vi "compareScan_Read.vi"() -> ()   [LabVIEW 2018]
uses:
  MotorController/#include/Global textParse.vi
panel:
  out "ILpass":bool=TRUE
  out "IRCpass":bool=TRUE
  out "Fpass":bool=TRUE
  out "ILimit":string
  out "IrComp":string
  out "Firmware":string
  out "Test":string
  in  "E-Stop":bool
  in  "Barcode Scan":string
  out "ScanNumber":string
  out "NumberMatch":bool
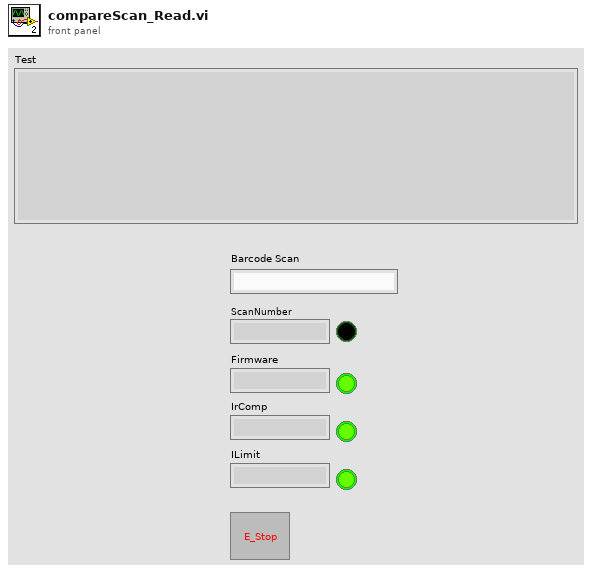
[diagram p1: front panel]
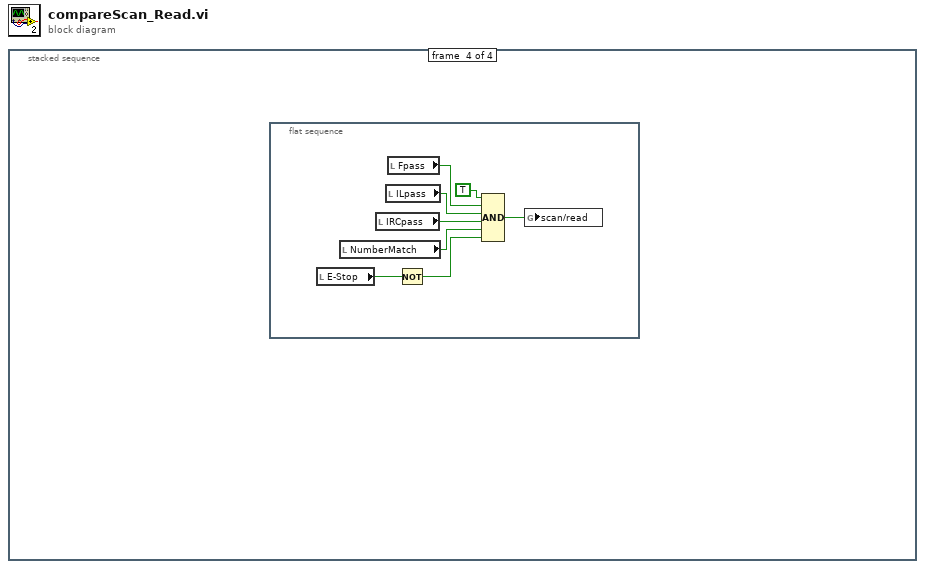
[diagram p0: block diagram]
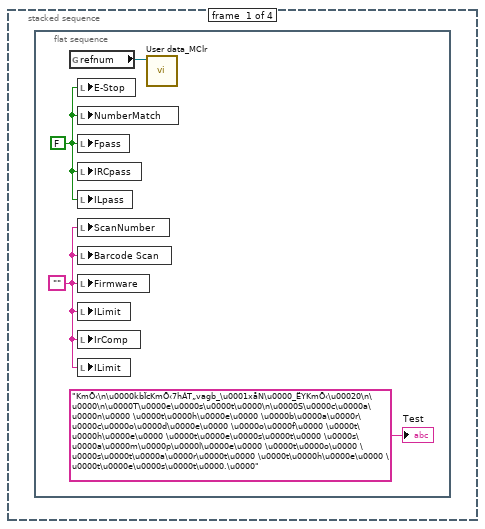
[diagram p2: hidden frame]
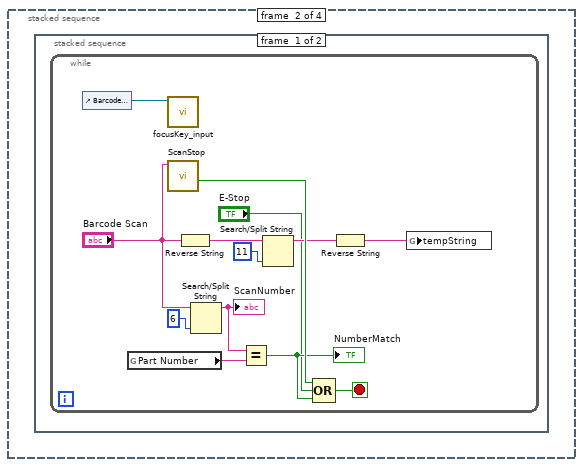
[diagram p3: hidden frame]
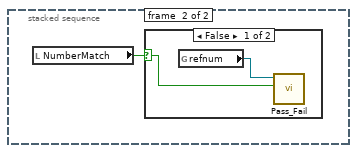
[diagram p4: hidden frame]
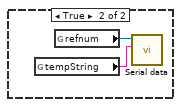
[diagram p5: hidden frame]
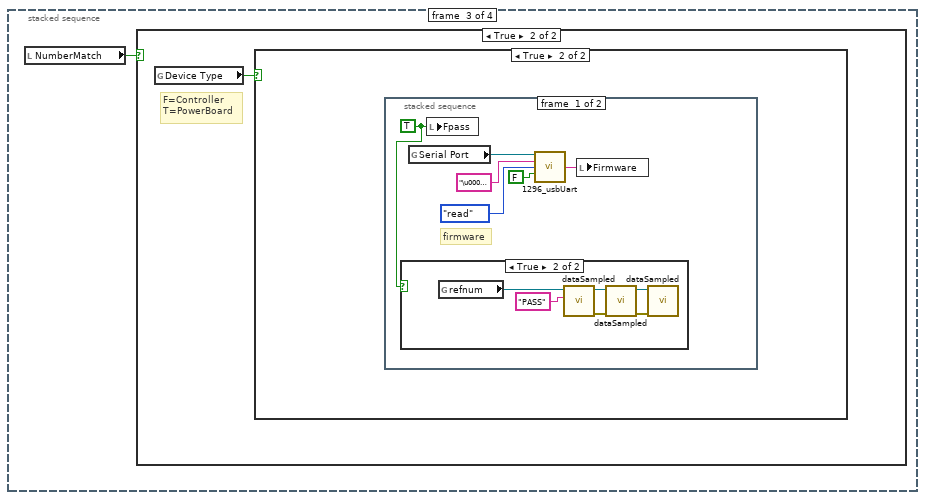
[diagram p6: hidden frame]
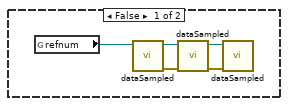
[diagram p7: hidden frame]
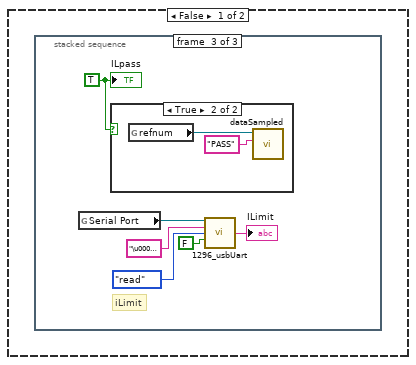
[diagram p8: hidden frame]
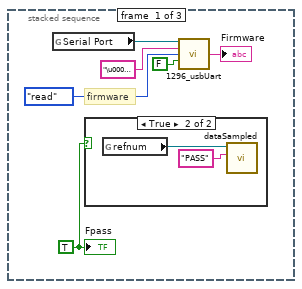
[diagram p9: hidden frame]
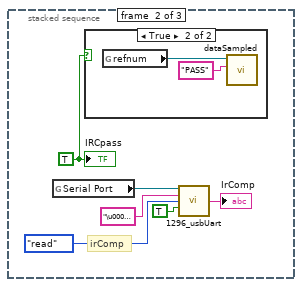
[diagram p11: hidden frame]
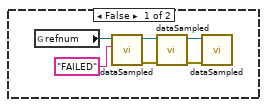
[diagram p14: hidden frame]
diagram:
  n1 = stacked-sequence {
    frame #0 {
      n2 = flat-sequence {
        frame #0 {
          w3 = FALSE
          w2 = ""
          n3 = global read "Global textParse.vi" "refnum"() -> (w4:refnum<file>)
          n4 = local write "E-Stop"(w3) -> ()
          n5 = local write "NumberMatch"(w3) -> ()
          n6 = local write "Fpass"(w3) -> ()
          n7 = local write "IRCpass"(w3) -> ()
          n8 = local write "ILpass"(w3) -> ()
          n9 = local write "ScanNumber"(w2) -> ()
          n10 = local write "Barcode Scan"(w2) -> ()
          n11 = local write "Firmware"(w2) -> ()
          n12 = local write "ILimit"(w2) -> ()
          n13 = local write "IrComp"(w2) -> ()
          n14 = local write "ILimit"(w2) -> ()
          n15 = call "User data_MClr.vi"("refnum in"=w4) -> ()  [unwired: 7 in, 2 out]
          "Test" <- "KmÕ‹\n\u0000kbÏcKmÕ‹7hÁT„vagb_\u0001xåN\u0000_ËYKmÕ‹\u00020\n\u0000\n\u0000T\u0000e\u0000s\u0000t\u0000\n\u0000S\u0000c\u0000a\u0000n\u0000 \u0000t\u0000h\u0000e\u0000 \u0000b\u0000a\u0000r\u0000c\u0000o\u0000d\u0000e\u0000 \u0000o\u0000f\u0000 \u0000t\u0000h\u0000e\u0000 \u0000t\u0000e\u0000s\u0000t\u0000 \u0000s\u0000a\u0000m\u0000p\u0000l\u0000e\u0000 \u0000t\u0000o\u0000 \u0000s\u0000t\u0000a\u0000r\u0000t\u0000 \u0000t\u0000h\u0000e\u0000 \u0000t\u0000e\u0000s\u0000t\u0000.\u0000"
        }
      }
    }
    frame #1 {
      n16 = stacked-sequence {
        frame #0 {
          n17 = while {
            stop <- w12 stop-if-true
            n18 = control-ref of="Barcode Scan"() -> (w17:refnum<vi>)
            n19 = global read "Global textParse.vi" "Part Number"() -> (w9:string)
            n20 = call "focusKey_input.vi"("reference"=w17) -> ()  [unwired: 10 in, 1 out]
            n21 = call "ScanStop.vi"("bar code scan"="Barcode Scan") -> ("Output"=w16:bool)  [unwired: 8 in, 2 out]
            n22 = Reverse String(1:"Barcode Scan") -> (0:w14:string)
            n23 = Search/Split String(string="Barcode Scan", offset (0)=6) -> (substring before match=w8:string)  [unwired: 1 in, 2 out]
            "ScanNumber" <- w8
            n24 = Equal?(x=w8, y=w9) -> (x = y?=w7:bool)
            "NumberMatch" <- w7
            n25 = Search/Split String(string=w14, offset (0)=11) -> (substring before match=w15:string)  [unwired: 1 in, 2 out]
            n26 = Compound Arithmetic op=OR(w16, "E-Stop", w7) -> (w12:bool)
            n27 = Reverse String(1:w15) -> (0:w6:string)
            n28 = global write "Global textParse.vi" "tempString"(w6) -> ()
          }
        }
        frame #1 {
          n29 = local read "NumberMatch"() -> (w18:bool)
          n30 = case shown="False" w18 {
            selector: w18 -> [w19 _]
            frame False {
              n31 = global read "Global textParse.vi" "refnum"() -> (w20:refnum<file>)
              n32 = call "Pass_Fail.vi"("OK"=w19, "Byte Stream File in"=w20) -> ()  [unwired: 8 in, 2 out]
            }
            frame True {
              n33 = global read "Global textParse.vi" "tempString"() -> (w22:string)
              n34 = global read "Global textParse.vi" "refnum"() -> (w21:refnum<file>)
              n35 = call "Serial data.vi"("Serial Number"=w22, "refnum in"=w21) -> ()  [unwired: 8 in, 2 out]
            }
          }
        }
      }
    }
    frame #2 {
      n36 = local read "NumberMatch"() -> (w23:bool)
      n37 = case shown="True" w23 {
        frame False {
          n38 = global read "Global textParse.vi" "refnum"() -> (w28:refnum<file>)
          n39 = call "dataSampled.vi"("refnum in"=w28) -> ("error out"=w27:errorcluster, "refnum out"=w26:refnum<file>)  [unwired: 9 in]
          n40 = call "dataSampled.vi"("Error In"=w27, "refnum in"=w26) -> ("error out"=w25:errorcluster, "refnum out"=w24:refnum<file>)  [unwired: 8 in]
          n41 = call "dataSampled.vi"("Error In"=w25, "refnum in"=w24) -> ()  [unwired: 8 in, 2 out]
        }
        frame True {
          # "F=Controller\nT=PowerBoard"
          n42 = global read "Global textParse.vi" "Device Type"() -> (w29:bool)
          n43 = case shown="True" w29 {
            frame False {
              n44 = stacked-sequence {
                frame #0 {
                  w30 = TRUE ("Fpass")
                  # "firmware"
                  n45 = global read "Global textParse.vi" "Serial Port"() -> (w35:refnum<visa-resource-name>)
                  n46 = case shown="True" w30 {
                    frame False {
                    }
                    frame True {
                      n47 = global read "Global textParse.vi" "refnum"() -> (w37:refnum<file>)
                      n48 = call "dataSampled.vi"("Data"="PASS", "refnum in"=w37) -> ()  [unwired: 8 in, 2 out]
                    }
                  }
                  n49 = call "1296_usbUart.vi"("VISA resource name"=w35, "command"="\u0005\u0002", "r/w"=enum16{"read", "write"}."read", "resetValues"=FALSE) -> ("byte[5]"=→"Firmware":string)  [unwired: 8 in, 3 out]
                  "Fpass" <- w30
                }
                frame #1 {
                  w38 = TRUE ("IRCpass")
                  # "irComp"
                  n50 = global read "Global textParse.vi" "Serial Port"() -> (w43:refnum<visa-resource-name>)
                  n51 = case shown="True" w38 {
                    frame False {
                    }
                    frame True {
                      n52 = global read "Global textParse.vi" "refnum"() -> (w45:refnum<file>)
                      n53 = call "dataSampled.vi"("Data"="PASS", "refnum in"=w45) -> ()  [unwired: 8 in, 2 out]
                    }
                  }
                  n54 = call "1296_usbUart.vi"("VISA resource name"=w43, "command"="\u0001\u0004", "r/w"=enum16{"read", "write"}."read", "resetValues"=TRUE) -> ("byte[5]"=→"IrComp":string)  [unwired: 8 in, 3 out]
                  "IRCpass" <- w38
                }
                frame #2 {
                  w46 = TRUE ("ILpass")
                  # "iLimit"
                  n55 = global read "Global textParse.vi" "Serial Port"() -> (w51:refnum<visa-resource-name>)
                  n56 = case shown="True" w46 {
                    frame False {
                    }
                    frame True {
                      n57 = global read "Global textParse.vi" "refnum"() -> (w53:refnum<file>)
                      n58 = call "dataSampled.vi"("Data"="PASS", "refnum in"=w53) -> ()  [unwired: 8 in, 2 out]
                    }
                  }
                  n59 = call "1296_usbUart.vi"("VISA resource name"=w51, "command"="\u0001\u0005", "r/w"=enum16{"read", "write"}."read", "resetValues"=FALSE) -> ("byte[5]"=→"ILimit":string)  [unwired: 8 in, 3 out]
                  "ILpass" <- w46
                }
              }
            }
            frame True {
              n60 = stacked-sequence {
                frame #0 {
                  w54 = TRUE ("Fpass")
                  # "firmware"
                  n61 = case shown="True" w54 {
                    frame False {
                      n62 = global read "Global textParse.vi" "refnum"() -> (w65:refnum<file>)
                      n63 = call "dataSampled.vi"("Data"="FAILED", "refnum in"=w65) -> ("error out"=w64:errorcluster, "refnum out"=w63:refnum<file>)  [unwired: 8 in]
                      n64 = call "dataSampled.vi"("Error In"=w64, "refnum in"=w63) -> ("error out"=w62:errorcluster, "refnum out"=w61:refnum<file>)  [unwired: 8 in]
                      n65 = call "dataSampled.vi"("Error In"=w62, "refnum in"=w61) -> ()  [unwired: 8 in, 2 out]
                    }
                    frame True {
                      n66 = global read "Global textParse.vi" "refnum"() -> (w71:refnum<file>)
                      n67 = call "dataSampled.vi"("Data"="PASS", "refnum in"=w71) -> ("error out"=w70:errorcluster, "refnum out"=w69:refnum<file>)  [unwired: 8 in]
                      n68 = call "dataSampled.vi"("Error In"=w70, "refnum in"=w69) -> ("error out"=w68:errorcluster, "refnum out"=w67:refnum<file>)  [unwired: 8 in]
                      n69 = call "dataSampled.vi"("Error In"=w68, "refnum in"=w67) -> ()  [unwired: 8 in, 2 out]
                    }
                  }
                  n70 = global read "Global textParse.vi" "Serial Port"() -> (w59:refnum<visa-resource-name>)
                  n71 = local write "Fpass"(w54) -> ()
                  n72 = call "1296_usbUart.vi"("VISA resource name"=w59, "command"="\u0005\u0002", "r/w"=enum16{"read", "write"}."read", "resetValues"=FALSE) -> ("byte[5]"=w55:string)  [unwired: 8 in, 3 out]
                  n73 = local write "Firmware"(w55) -> ()
                }
                frame #1 {
                }
              }
            }
          }
        }
      }
    }
    frame #3 {
      n74 = flat-sequence {
        frame #0 {
          n75 = local read "E-Stop"() -> (w77:bool)
          n76 = local read "NumberMatch"() -> (w76:bool)
          n77 = local read "IRCpass"() -> (w75:bool)
          n78 = local read "ILpass"() -> (w74:bool)
          n79 = local read "Fpass"() -> (w73:bool)
          n80 = Not(x=w77) -> (.not. x?=w78:bool)
          n81 = Compound Arithmetic op=AND(TRUE ("value"), w73, w74, w75, w76, w78) -> (w79:bool)
          n82 = global write "Global textParse.vi" "scan/read"(w79) -> ()
        }
      }
    }
  }
